vi "Status Channels Get reference and sort.vi"(8 "error in (no error)":errorcluster, 11 "Item Ref":T1 format="%.0x") -> (0 "error out":errorcluster, 3 "Channel Refs":T1[](array[typedef]) format="%.0x")   [LabVIEW 2020, in "Shared Variables CD 2.0 Engine.lvlib"]
uses:
  Shared Variables CD 2.0 Engine.lvlib
  <vilib>/NI VeriStand/Custom Device Tools/Custom Device Utility Library/Custom Device Utility Library.lvlib
  <vilib>/NI VeriStand/Custom Device API/Custom Device API.lvlib
  Shared/SV Global.vi
  <vilib>/NI VeriStand/Custom Device API/Custom Device Item Ref.ctl
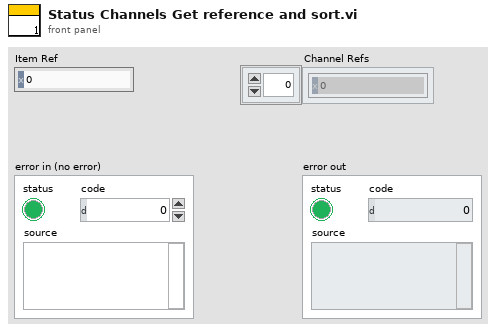
[diagram p1: front panel]
types:
  T1 = typedef "Custom Device API.lvlib/Custom Device Item Ref.ctl" = u64
  T2 = typedef "Custom Device API.lvlib/Custom Device Item Info.ctl" = cluster{"Name":string, "Is Channel":bool, "GUID":string, "Is Waveform":bool}
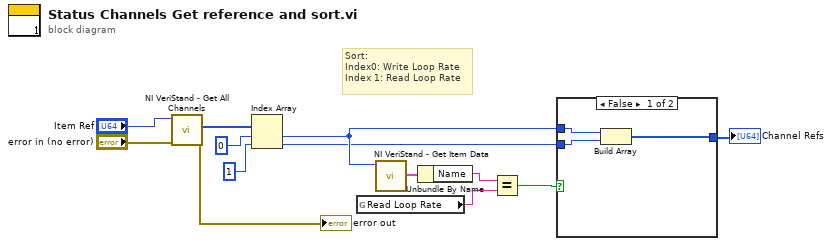
[diagram p0: block diagram]
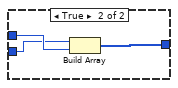
[diagram p2: hidden frame]
diagram:
  # "Sort:\nIndex0: Write Loop Rate\nIndex 1: Read Loop Rate"
  n1 = call <vilib>:"NI VeriStand - Get All Channels.vi"("error in"="error in (no error)", "Section Ref in"="Item Ref") -> ("error out"=→"error out":errorcluster, "Channel Refs"=w10:T1[])  [unwired: 6 in, 2 out]
  n2 = Index Array(array=w10, index #1=0 ("index"), index #2=1 ("index")) -> (element #1=w3:T1, element #2=w2:T1)
  n3 = global read "SV Global.vi" "Read Loop Rate"() -> (w5:string)
  n4 = call <vilib>:"NI VeriStand - Get Item Data.vi"("Item Ref in"=w3) -> ("Item Info"=w7:T2)  [unwired: 7 in, 3 out]
  n5 = Unbundle By Name(w7) -> ("Name"=w6:string)
  n6 = Equal?(x=w6, y=w5) -> (x = y?=w4:bool)
  n7 = case shown="False" w4 {
    tunnel: w3 -> [w16 w19]
    tunnel: w2 -> [w15 w18]
    tunnel: [w14 w17] -> w1
    frame False {
      n8 = Build Array(w16, w15) -> (w14:T1[])
    }
    frame True {
      n9 = Build Array(w18, w19) -> (w17:T1[])
    }
  }
  "Channel Refs" <- w1
